vi "Curtin1_Color.vi"(8 "Offset":u16, 10 "Files in":T1[](array[typedef]), 11 "Color":u32[](array[colorbox])) -> (2 "New color":u32, 3 "Color palette":u32[](array[colorbox]))   [LabVIEW 2022 SP3]
uses:
  Curtin1_Label.ctl
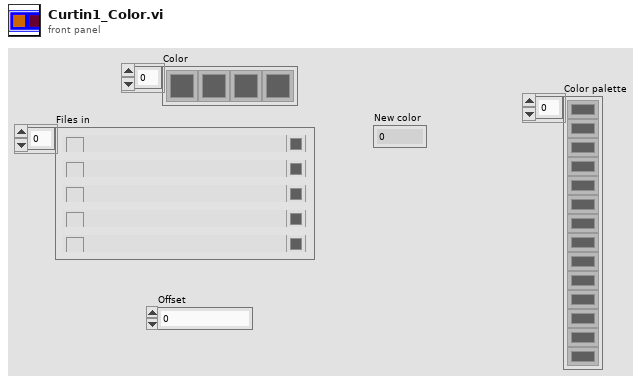
[diagram p1: front panel]
types:
  T1 = typedef "Curtin1_Label.ctl" = cluster{"Show?":bool, "Name":string, "Color":u32, "Path":path, "Show Notes":bool}
  T2 = enum16{"big-endian, network order", "native, host order", "little-endian"}
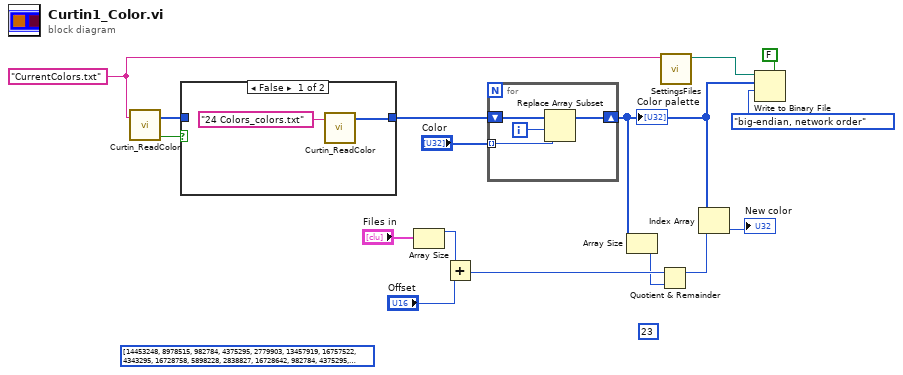
[diagram p0: block diagram]
diagram:
  (unwired) 23 ("y")
  w2 = "CurrentColors.txt" ("name or relative path")
  (unwired) u32[] [14453248, 8978515, 982784, 4375295, 2779903, 13457919, 16757522, 4343295, 16728758, 5898228, 2838827, 16728642, 982784, 4375295, 13827953, 13457919, 16757522, 4343295, 16728758, 5898228, 16777215, 16728642, 982784, 4375295, 13827953, 13457919, 16757522, 4343295, 16728758, 5898228, 16777215, 16728642, 982784, 4375295, 13827953, 13457919, 16757522, 4343295, 16728758, 5898228, 16777215, 16728642, 982784, 4375295, 13827953, 13457919, 16757522, 4343295, 16728758, 5898228, 16777215, 16728642, 982784, 4375295, 13827953, 13457919, 16757522, 4343295, 16728758, 5898228, 16777215, 16728642, 982784, 4375295, 13827953, 13457919, 16757522, 4343295, 16728758, 5898228, 16777215, 16728642, 982784, 4375295, 13827953, 13457919, 16757522, 4343295, 16728758, 5898228, 16777215, 16728642, 982784, 4375295, 13827953, 13457919, 16757522, 4343295, 16728758, 5898228, 16777215, 16728642, 982784, 4375295, 13827953, 13457919, 16757522, 4343295, 16728758, 5898228] ("Array")
  n1 = call "Curtin_ReadColor.vi"("color file name"=w2) -> ("Success?"=w5:bool, "Colors"=w4:u32[])  [unwired: 1 in]
  n2 = case shown="False" w5 {
    tunnel: [w17 w19] -> w3
    tunnel: w4 -> [_ w19]
    frame False {
      n3 = call "Curtin_ReadColor.vi"("color file name"="24 Colors_colors.txt" ("name or relative path")) -> ("Colors"=w17:u32[])  [unwired: 1 in, 1 out]
    }
    frame True {
    }
  }
  n4 = Array Size(array="Files in") -> (size(s)=w13:i32)
  n5 = Add(x=w13, y="Offset") -> (x+y=w12:i32)
  n6 = for {
    shift-right: [w22] -> w8
    shift-left: w3 -> [w23]
    tunnel: "Color" -> [w20] mode=indexing
    i -> [w21]
    n7 = Replace Array Subset(array=w23, new element=w20, index=w21) -> (w22:u32[])
  }
  "Color palette" <- w8
  n8 = Array Size(array=w8) -> (size(s)=w7:i32)
  n9 = Quotient & Remainder(x=w12, y=w7) -> (x-y*floor(x/y)=w11:i32)  [unwired: 1 out]
  n10 = call "SettingsFiles.vi"("settings file name"=w2) -> ("file path"=w1:path)  [unwired: 9 in, 1 out]
  n11 = Index Array(array=w8, index=w11) -> (element=→"New color":u32)
  n12 = Write to Binary File(file (use dialog)=w1, data=w8, 5:FALSE ("prepend array or string size? (T)"), 9:T2."big-endian, network order" ("byte order (0:big-endian, network order)")) -> ()  [unwired: 2 in, 3 out]
